vi "DelayProject_AirDelay.vi"() -> ()   [LabVIEW 2020]
uses:
  C:/DATA/Megan/LabviewScripts/ThorlabsKinesisDrivers/Thorlabs.MotionControl.Benchtop.BrushlessMotorCLI.dll
  Thorlabs.MotionControl.Benchtop.BrushlessMotorCLI.dll
  C:/DATA/Megan/LabviewScripts/ThorlabsKinesisDrivers/Thorlabs.MotionControl.Controls.dll
  Thorlabs.MotionControl.Controls.dll
  Program Files (x86)/National Instruments/LabVIEW 2011/user.lib/Nanonis Prog Interface/Nanonis Prog Interface.lvlib
panel:
  in  "Start Move B":bool
  in  "Set Position B (mm)":ext format="%.3f"
  in  "Clear Plots":bool
  in  "Data3":dbl[][](array[numeric])
  out "AFM":cluster{dbl[], dbl[]}[](graph)
  in  "Data2":dbl[][](array[numeric])
  in  "Data1":dbl[][](array[numeric])
  in  "Plot3":bool
  in  "Plot2":bool
  in  "Plot1":bool
  out "Optics":cluster{dbl[], dbl[]}[](graph)
  out "Array":string[][](array[string])
  in  "AC bias (Hz)":string
  in  "AC bias":string
  in  "DC bias":string
  in  "Tip lift":string
  in  "Time const":string
  in  "Prop gain":string
  in  "Polarization":string
  in  "Notes":string
  in  "Location":string
  out "AC bias (Hz)":string="AC Bias (Hz)"
  out "AC bias":string="AC Bias (V)"
  out "DC bias":string="DC Bias (V)"
  out "Polarization":string="Polarization (deg)"
  out "Tip Lift":string="Tip Lift"
  out "Notes":string="Notes"
  out "Location":string="Location"
  out "Time Const":string="Time constant (s)"
  out "Prop Gain":string="Proportional gain (m/Hz)"
  in  "Net Power":string
  in  "Wavelength":string
  out "Net Power":string="Net power (mW)"
  out "Wavelength":string="Wavelength (nm)"
  out "Instantaneous":dbl
  in  "Channel":dbl
  out "Average":dbl
  in  "Wait After (ms)":dbl=100.0
  in  "Wait Before (ms)":dbl=100.0
  in  "Points per Step":dbl=10.0
  in  "Save Sweep":bool
  out "Total Time (min:sec)":string
  out "Range (fs)":dbl
  out "Total Distance (mm)":dbl
  in  "Step Size (mm)":dbl format="%.4f"
  in  "Start Position (mm)":dbl=80.0
  in  "End Position (mm)":dbl=90.0
  out "Step Size (fs)":dbl=100.0
  out "Status":string
  in  "Set Position A (mm)":ext format="%.3f"
  in  "Start Move A":bool
  in  "Start Sweep":bool
  out "Time Remaining (min:sec)":string
  in  "Stop Sweep":bool
  out "Position  (mm)":ext format="%.3f"
  in  "BenchtopBrushlessControl":refnum<k24>(container)
  # "Air Delay"
  # "Sweep"
  # "This program moves the DSS022 translational delay stage either in a single step (Move), or a  stepped sweep (Sweep). \n\nThe sequence of events in the Sweep is as follows:\n1) Home the stage.\n2) Go to the Start Position; wait 1s.\n3) Move by Step Size.\n4)  Wait Before time. \n5) Write Position to Nanonis Output 8.\n6) Read all Nanonis Channels, Points per Step times.\n7) Take the average of these instantaneous readouts.\n8) Wait After time.\n9) Repeat 3-8 for each step. \n10) Save all Nanonis channels and record Attributes in header.\n\nThe Readouts are for this VI display only, to visualize what the program is doing. Channel is the Nanonis channel displayed. \n\nIf the Set/Start/End positions are outside of the operating range [50:210]mm, the Move/Sweep will not execute. Short wait times may lead to errors if  they don't allow time  to move. \n\nThis VI needs to be opened from the project directory. This project and VI need to be in the same directory as the Thorlabs Kinesis folder, and require a 64-bit version of Labview. This program cannot run simultaneously with WedgeDelay.vi"
  # "Attributes"
  # "Parameters"
  # "Readouts"
  # "Move A"
  # "Move B"
  # "Wedge Delay: 43mm"
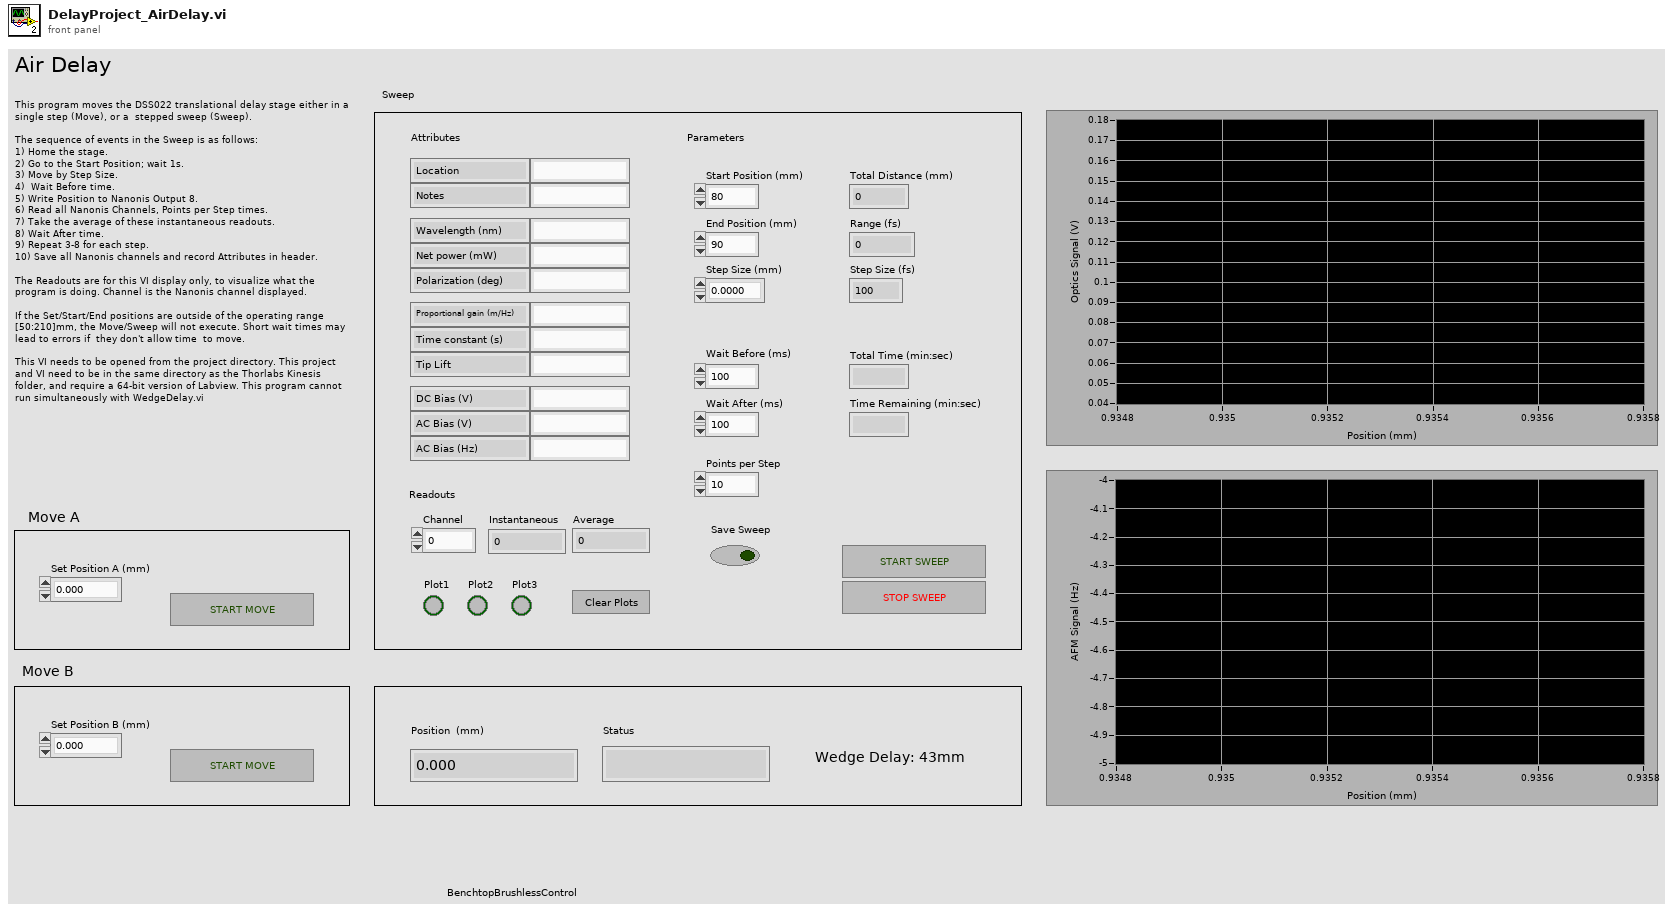
[diagram p1: front panel]
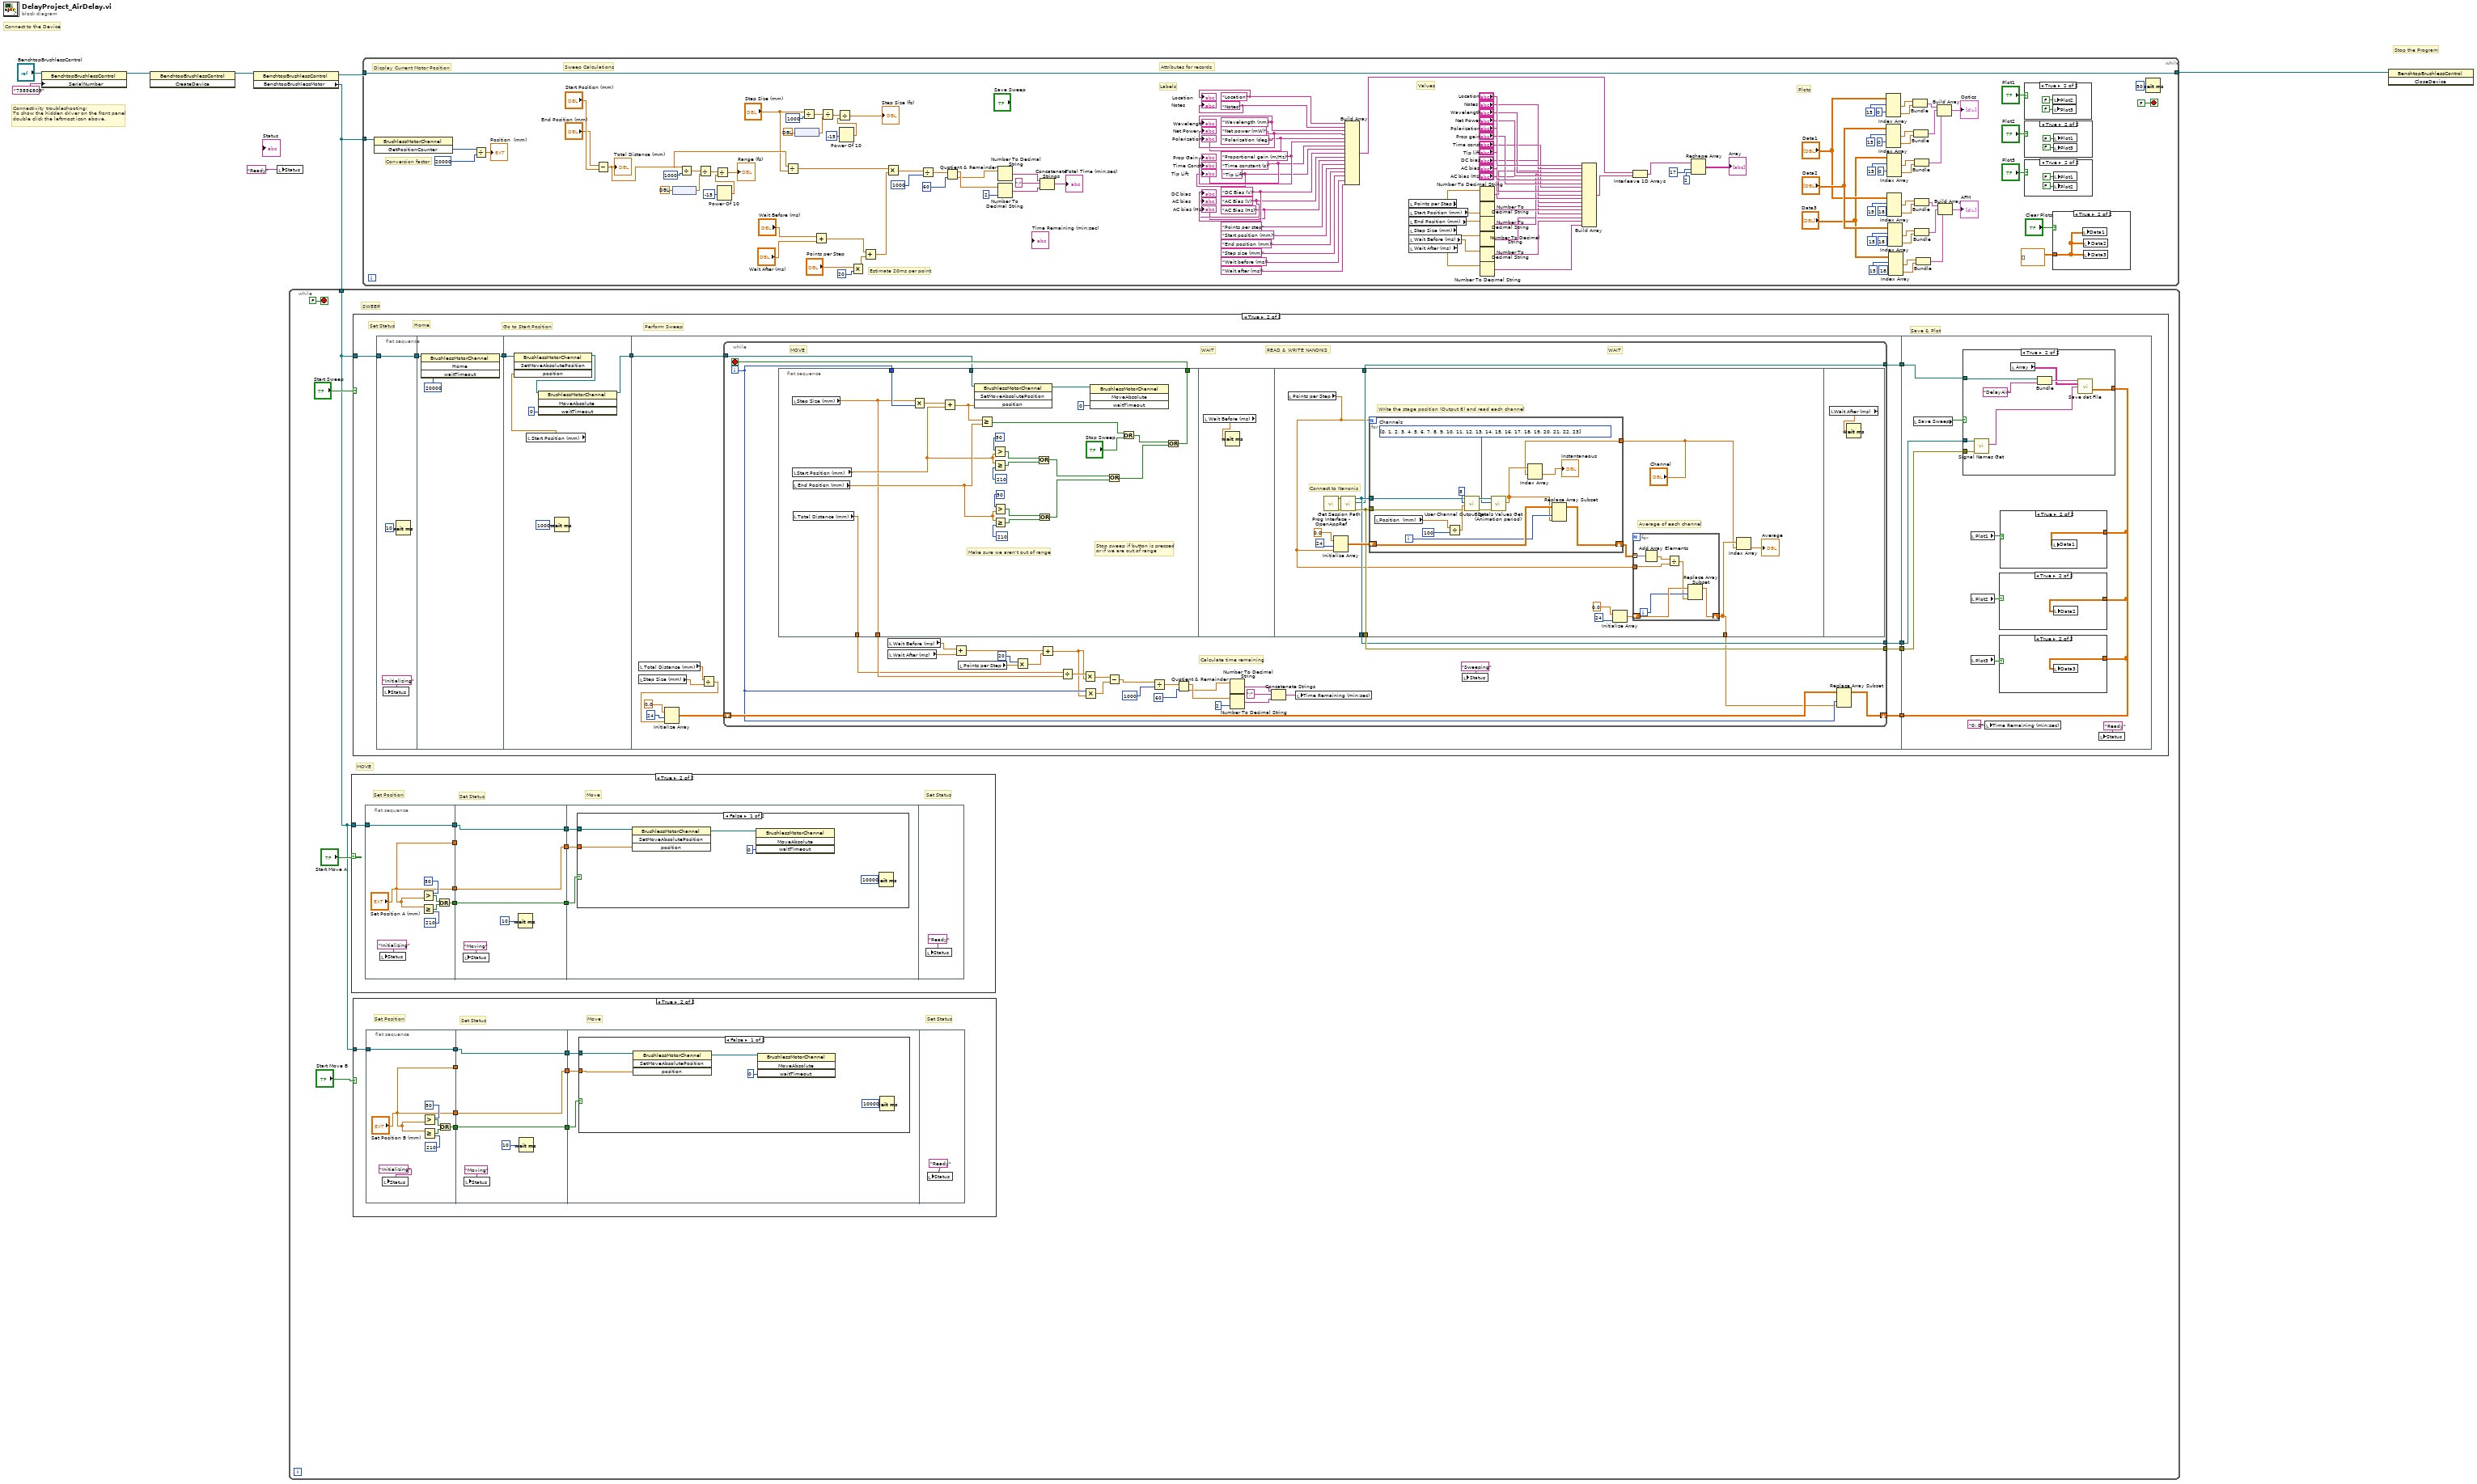
[diagram p0: block diagram]
diagram:
  # "Connectivity troubleshooting: \nTo show the hidden driver on the front panel \ndouble click the leftmost icon above."
  # "Stop the Program"
  # "Connect to the Device"
  n1 = property class="BenchtopBrushlessControl"(reference="BenchtopBrushlessControl", "SerialNumber"="73856809") -> (reference out=w7:refnum<k24>)  [unwired: 1 in, 1 out]
  n2 = invoke class="BenchtopBrushlessControl" method="CreateDevice"(reference=w7) -> (reference out=w4:refnum<k24>)  [unwired: 2 in, 2 out]
  n3 = property class="BenchtopBrushlessControl"(reference=w4) -> (reference out=w3:refnum<k24>, "BenchtopBrushlessMotor"=w2:refnum<k24>)  [unwired: 1 in, 1 out]
  n4 = local write "Status"("Ready") -> ()
  n5 = while {
    tunnel: w2 -> [w9]
    stop <- FALSE stop-if-true
    # "MOVE"
    # "SWEEP"
    n6 = case shown="True" "Start Move A" {
      tunnel: w9 -> [_ w51]
      frame False {
      }
      frame True {
        # "Set Status"
        # "Move"
        # "Set Status"
        # "Set Position"
        n7 = flat-sequence {
          tunnel: w51 -> [w59]
          tunnel: [w59] -> w50
          tunnel: ["Set Position A (mm)"] -> w49
          tunnel: [w53] -> w48
          tunnel: ["Set Position A (mm)"] -> w45
          tunnel: w50 -> [w62]
          tunnel: w49 -> [_]
          tunnel: w48 -> [w64]
          tunnel: [w64] -> w47
          tunnel: [w63] -> w46
          tunnel: w45 -> [w63]
          tunnel: [w62] -> w44
          tunnel: w47 -> [w67]
          tunnel: w46 -> [w66]
          tunnel: w44 -> [w65]
          frame #0 {
            n8 = local write "Status"("Initializing") -> ()
            n9 = Greater?(x=50, y="Set Position A (mm)") -> (0:w58:bool)
            n10 = Greater Or Equal?(x="Set Position A (mm)", y=210) -> (x >= y?=w57:bool)
            n11 = Or(x=w58, y=w57) -> (x .or. y?=w53:bool)
          }
          frame #1 {
            n12 = local write "Status"("Moving") -> ()
            n13 = Wait (ms)(milliseconds to wait=10) -> ()  [unwired: 1 out]
          }
          frame #2 {
            n14 = case shown="False" w67 {
              tunnel: w66 -> [w69 _]
              tunnel: w65 -> [w70 _]
              frame False {
                n15 = invoke class="BrushlessMotorChannel" method="SetMoveAbsolutePosition"(reference=w70, "position"=w69) -> (reference out=w72:refnum<k24>)  [unwired: 2 in, 3 out]
                n16 = invoke class="BrushlessMotorChannel" method="MoveAbsolute"(reference=w72, "waitTimeout"=0) -> ()  [unwired: 2 in, 4 out]
                n17 = Wait (ms)(milliseconds to wait=10000) -> ()  [unwired: 1 out]
              }
              frame True {
              }
            }
          }
          frame #3 {
            n18 = local write "Status"("Ready") -> ()
          }
        }
      }
    }
    n19 = case shown="True" "Start Move B" {
      tunnel: w9 -> [_ w21]
      frame False {
      }
      frame True {
        # "Set Status"
        # "Move"
        # "Set Status"
        # "Set Position"
        n20 = flat-sequence {
          tunnel: w21 -> [w29]
          tunnel: [w29] -> w20
          tunnel: ["Set Position B (mm)"] -> w19
          tunnel: [w24] -> w18
          tunnel: ["Set Position B (mm)"] -> w15
          tunnel: w20 -> [w32]
          tunnel: w19 -> [_]
          tunnel: w18 -> [w34]
          tunnel: [w34] -> w17
          tunnel: [w33] -> w16
          tunnel: w15 -> [w33]
          tunnel: [w32] -> w14
          tunnel: w17 -> [w37]
          tunnel: w16 -> [w36]
          tunnel: w14 -> [w35]
          frame #0 {
            n21 = local write "Status"("Initializing") -> ()
            n22 = Greater?(x=50, y="Set Position B (mm)") -> (0:w28:bool)
            n23 = Greater Or Equal?(x="Set Position B (mm)", y=210) -> (x >= y?=w27:bool)
            n24 = Or(x=w28, y=w27) -> (x .or. y?=w24:bool)
          }
          frame #1 {
            n25 = local write "Status"("Moving") -> ()
            n26 = Wait (ms)(milliseconds to wait=10) -> ()  [unwired: 1 out]
          }
          frame #2 {
            n27 = case shown="False" w37 {
              tunnel: w36 -> [w39 _]
              tunnel: w35 -> [w40 _]
              frame False {
                n28 = invoke class="BrushlessMotorChannel" method="SetMoveAbsolutePosition"(reference=w40, "position"=w39) -> (reference out=w42:refnum<k24>)  [unwired: 2 in, 3 out]
                n29 = invoke class="BrushlessMotorChannel" method="MoveAbsolute"(reference=w42, "waitTimeout"=0) -> ()  [unwired: 2 in, 4 out]
                n30 = Wait (ms)(milliseconds to wait=10000) -> ()  [unwired: 1 out]
              }
              frame True {
              }
            }
          }
          frame #3 {
            n31 = local write "Status"("Ready") -> ()
          }
        }
      }
    }
    n32 = case shown="True" "Start Sweep" {
      tunnel: w9 -> [_ w81]
      frame False {
      }
      frame True {
        # "Save & Plot"
        # "Set Status"
        # "Perform Sweep"
        # "Go to Start Position"
        # "Home"
        n33 = flat-sequence {
          tunnel: w81 -> [w84]
          tunnel: [w84] -> w80
          tunnel: [w85] -> w79
          tunnel: w80 -> [w87]
          tunnel: w79 -> [w93]
          tunnel: [w90] -> w78
          tunnel: w78 -> [w104]
          tunnel: [w103] -> w77
          tunnel: [w102] -> w76
          tunnel: [w101] -> w75
          tunnel: [w94] -> w74
          tunnel: w77 -> [w210]
          tunnel: w76 -> [w209]
          tunnel: w75 -> [w208]
          tunnel: w74 -> [w206]
          frame #0 {
            n34 = local write "Status"("Initializing") -> ()
            n35 = Wait (ms)(milliseconds to wait=10) -> ()  [unwired: 1 out]
          }
          frame #1 {
            n36 = invoke class="BrushlessMotorChannel" method="Home"(reference=w87, "waitTimeout"=20000) -> (reference out=w85:refnum<k24>)  [unwired: 2 in, 3 out]
          }
          frame #2 {
            n37 = local read "Start Position (mm)"() -> (w88:dbl)
            n38 = invoke class="BrushlessMotorChannel" method="SetMoveAbsolutePosition"(reference=w93, "position"=w88) -> (reference out=w91:refnum<k24>)  [unwired: 2 in, 3 out]
            n39 = invoke class="BrushlessMotorChannel" method="MoveAbsolute"(reference=w91, "waitTimeout"=0) -> (reference out=w90:refnum<k24>)  [unwired: 2 in, 3 out]
            n40 = Wait (ms)(milliseconds to wait=1000) -> ()  [unwired: 1 out]
          }
          frame #3 {
            n41 = local read "Step Size (mm)"() -> (w97:dbl)
            n42 = local read "Total Distance (mm)"() -> (w98:dbl)
            n43 = Divide(x=w98, y=w97) -> (x/y=w96:dbl)
            n44 = Initialize Array(0.0, 24, w96) -> (w95:dbl[][])
            n45 = while {
              tunnel: w104 -> [w136]
              tunnel: [w116] -> w103
              tunnel: [w117] -> w102
              tunnel: [w115] -> w101
              shift-right: [w111] -> w94
              shift-left: w95 -> [w114]
              i -> [w113]
              stop <- w137 stop-if-true
              # "WAIT"
              # "READ & WRITE NANONIS"
              # "WAIT"
              # "MOVE"
              # "Calculate time remaining"
              n46 = flat-sequence {
                tunnel: w113 -> [w142]
                tunnel: [w141] -> w137
                tunnel: w136 -> [w140]
                tunnel: [w139] -> w126
                tunnel: [w138] -> w125
                tunnel: [w169] -> w117
                tunnel: [w168] -> w116
                tunnel: [w167] -> w115
                tunnel: [w166] -> w112
                frame #0 {
                  # "Stop sweep if button is pressed\nor if we are out of range"
                  # "Make sure we aren't out of range"
                  n47 = local read "Step Size (mm)"() -> (w139:dbl)
                  n48 = local read "Start Position (mm)"() -> (w161:dbl)
                  n49 = local read "End Position (mm)"() -> (w162:dbl)
                  n50 = local read "Total Distance (mm)"() -> (w138:dbl)
                  n51 = Multiply(x=w139, y=w142) -> (x*y=w147:dbl)
                  n52 = Add(x=w147, y=w161) -> (x+y=w148:dbl)
                  n53 = invoke class="BrushlessMotorChannel" method="SetMoveAbsolutePosition"(reference=w140, "position"=w148) -> (reference out=w143:refnum<k24>)  [unwired: 2 in, 3 out]
                  n54 = Greater Or Equal?(x=w148, y=w162) -> (x >= y?=w146:bool)
                  n55 = Greater?(x=50, y=w161) -> (0:w153:bool)
                  n56 = Greater Or Equal?(x=w161, y=210) -> (x >= y?=w154:bool)
                  n57 = Greater?(x=50, y=w162) -> (0:w157:bool)
                  n58 = Greater Or Equal?(x=w162, y=210) -> (x >= y?=w158:bool)
                  n59 = Or(x=w153, y=w154) -> (x .or. y?=w159:bool)
                  n60 = Or(x=w157, y=w158) -> (x .or. y?=w160:bool)
                  n61 = invoke class="BrushlessMotorChannel" method="MoveAbsolute"(reference=w143, "waitTimeout"=0) -> ()  [unwired: 2 in, 4 out]
                  n62 = Or(x=w159, y=w160) -> (x .or. y?=w150:bool)
                  n63 = Or(x=w146, y="Stop Sweep") -> (x .or. y?=w149:bool)
                  n64 = Or(x=w149, y=w150) -> (x .or. y?=w141:bool)
                }
                frame #1 {
                  n65 = local read "Wait Before (ms)"() -> (w163:dbl)
                  n66 = Wait (ms)(milliseconds to wait=w163) -> ()  [unwired: 1 out]
                }
                frame #2 {
                  # "Write the stage position (Output 8) and read each channel"
                  # "Average of each channel"
                  # "Connect to Nanonis"
                  n67 = local read "Points per Step"() -> (w165:dbl)
                  n68 = call "Prog Interface - OpenAppRef.vi"() -> ("Error out"=w170:errorcluster, "Application reference"=w171:refnum<vi>)  [unwired: 6 in]
                  n69 = Initialize Array(0.0, 24, w165) -> (w174:dbl[][])
                  n70 = call "Get Session Path.vi"("error in (no error)"=w170, "Application ref in"=w171) -> ("error out"=w169:errorcluster, "Session path"=w167:path, "Application ref out"=w168:refnum<vi>)  [unwired: 7 in]
                  n71 = for {
                    N: w165 -> [_]
                    tunnel: w169 -> [w195]
                    tunnel: w168 -> [w194]
                    shift-right: [w193] -> w178
                    shift-left: w174 -> [w192]
                    tunnel: "Channel" -> [w187]
                    i -> [w191]
                    w188 = i32[] [0, 1, 2, 3, 4, 5, 6, 7, 8, 9, 10, 11, 12, 13, 14, 15, 16, 17, 18, 19, 20, 21, 22, 23]  # Channels
                    n72 = local read "Position  (mm)"() -> (w189:ext)
                    n73 = Divide(x=w189, y=100) -> (x/y=w198:ext)
                    n74 = call "User Channel Output Set.vi"("error in (no error)"=w195, "Output value (physical unit)"=w198, "User output channel (1-8)"=8, "Application ref in"=w194) -> ("error out"=w200:errorcluster, "Application ref out"=w199:refnum<vi>)  [unwired: 5 in]
                    n75 = call "Signals Values Get (Animation period).vi"("error in (no error)"=w200, "Signals indexes (0-23)"=w188, "Application ref in"=w199) -> ("Signals Values"=w190:sgl[])  [unwired: 5 in, 2 out]
                    n76 = Index Array(array=w190, index #1=w187) -> (element #1=→"Instantaneous":sgl)  [unwired: 1 in, 1 out]
                    n77 = Replace Array Subset(array=w192, new element=w190, index (col)=w191) -> (w193:dbl[][])  [unwired: 1 in]
                  }
                  n78 = Initialize Array(0.0, 24) -> (w177:dbl[])
                  n79 = for {
                    tunnel: w165 -> [w186]
                    tunnel: w178 -> [w182] mode=indexing
                    shift-right: [w184] -> w166
                    shift-left: w177 -> [w185]
                    i -> [w183]
                    n80 = Add Array Elements(numeric array=w182) -> (sum=w180:dbl)
                    n81 = Divide(x=w180, y=w186) -> (x/y=w181:dbl)
                    n82 = Replace Array Subset(array=w185, new element=w181, index=w183) -> (w184:dbl[])
                  }
                  n83 = Index Array(array=w166, index="Channel") -> (element=→"Average":dbl)
                }
                frame #3 {
                  n84 = local read "Wait After (ms)"() -> (w202:dbl)
                  n85 = Wait (ms)(milliseconds to wait=w202) -> ()  [unwired: 1 out]
                }
              }
              n86 = local read "Wait Before (ms)"() -> (w119:dbl)
              n87 = local read "Wait After (ms)"() -> (w118:dbl)
              n88 = Add(x=w119, y=w118) -> (x+y=w109:dbl)
              n89 = local read "Points per Step"() -> (w110:dbl)
              n90 = Multiply(x=20, y=w110) -> (x*y=w107:dbl)
              n91 = Add(x=w109, y=w107) -> (x+y=w108:dbl)
              n92 = Divide(x=w125, y=w126) -> (x/y=w127:dbl)
              n93 = Multiply(x=w127, y=w108) -> (x*y=w128:dbl)
              n94 = Multiply(x=w113, y=w108) -> (x*y=w130:dbl)
              n95 = Subtract(x=w128, y=w130) -> (x-y=w129:dbl)
              n96 = Divide(x=w129, y=1000) -> (x/y=w135:dbl)
              n97 = Quotient & Remainder(x=w135, y=60) -> (x-y*floor(x/y)=w134:dbl, floor(x/y)=w133:dbl)
              n98 = Number To Decimal String(number=w133) -> (decimal integer string=w132:string)  [unwired: 1 in]
              n99 = Number To Decimal String(number=w134, width (-)=2) -> (decimal integer string=w131:string)
              n100 = Concatenate Strings(w132, ":", w131) -> (w105:string)
              n101 = local write "Time Remaining (min:sec)"(w105) -> ()
              n102 = local write "Status"("Sweeping") -> ()
              n103 = Replace Array Subset(array=w114, new element=w112, index (col)=w113) -> (w111:dbl[][])  [unwired: 1 in]
            }
          }
          frame #4 {
            n104 = local read "Save Sweep"() -> (w211:bool)
            n105 = case shown="True" w211 {
              tunnel: w209 -> [_ w221]
              tunnel: w210 -> [_ w220]
              tunnel: w208 -> [_ w218]
              tunnel: w206 -> [_ w217]
              frame False {
              }
              frame True {
                n106 = call "Signal Names Get.vi"("error in (no error)"=w221, "Application ref in"=w220) -> ("Signals Names"=w219:string[])  [unwired: 5 in, 2 out]
                n107 = local read "Array"() -> (w216:string[][])
                n108 = Bundle("Session path"=w218, "DelayAir") -> (w223:cluster{"Session path":path, string})  [unwired: 1 in]
                n109 = call "Save dat File.vi"("Filename control"=w223, "Attributes"=w216, "Channels names"=w219, "Data"=w217) -> ()  [unwired: 8 in, 4 out]
              }
            }
            n110 = local read "Plot1"() -> (w203:bool)
            n111 = local read "Plot2"() -> (w204:bool)
            n112 = local read "Plot3"() -> (w205:bool)
            n113 = local write "Time Remaining (min:sec)"("0: 0") -> ()
            n114 = case shown="True" w204 {
              tunnel: w206 -> [_ w214]
              frame False {
              }
              frame True {
                n115 = local write "Data2"(w214) -> ()
              }
            }
            n116 = case shown="True" w205 {
              tunnel: w206 -> [_ w213]
              frame False {
              }
              frame True {
                n117 = local write "Data3"(w213) -> ()
              }
            }
            n118 = case shown="True" w203 {
              tunnel: w206 -> [_ w215]
              frame False {
              }
              frame True {
                n119 = local write "Data1"(w215) -> ()
              }
            }
            n120 = local write "Status"("Ready") -> ()
          }
        }
      }
    }
  }
  n121 = while {
    tunnel: [w355] -> w6
    tunnel: w3 -> [w355]
    tunnel: w2 -> [w354]
    stop <- FALSE stop-if-true
    w277 = "Polarization (deg)"
    w280 = "Notes"
    w281 = "Location"
    w274 = "Tip Lift"
    w271 = "AC Bias (Hz)"
    w272 = "AC Bias (V)"
    w273 = "DC Bias (V)"
    w275 = "Time constant (s)"
    w276 = "Proportional gain (m/Hz)"
    w278 = "Net power (mW)"
    w279 = "Wavelength (nm)"
    # "Plots"
    # "Estimate 20ms per point"
    # "Values"
    # "Labels"
    # "Attributes for records"
    # "Sweep Calculations"
    # "Display Current Motor Position"
    # "Conversion factor"
    n122 = invoke class="BrushlessMotorChannel" method="GetPositionCounter"(reference=w354) -> ("GetPositionCounter"=w353:i32)  [unwired: 2 in, 2 out]
    n123 = Divide(x=w353, y=20000) -> (x/y=→"Position  (mm)":dbl)
    n124 = Subtract(x="End Position (mm)", y="Start Position (mm)") -> (x-y=w321:dbl)
    "Total Distance (mm)" <- w321
    n125 = node(ext[unit] 299792458.0) -> (w337:ext)
    n126 = Divide(x=w321, y=1000) -> (x/y=w338:dbl)
    n127 = Divide(x=w338, y=w337) -> (x/y=w336:ext)
    n128 = Power Of 10(x=-15) -> (10^x=w333:dbl)
    n129 = Divide(x=w336, y=w333) -> (x/y=→"Range (fs)":ext)
    n130 = Divide(x=w321, y="Step Size (mm)") -> (x/y=w318:dbl)
    n131 = node(ext[unit] 299792458.0) -> (w347:ext)
    n132 = Divide(x="Step Size (mm)", y=1000) -> (x/y=w346:dbl)
    n133 = Add(x="Wait Before (ms)", y="Wait After (ms)") -> (x+y=w269:dbl)
    n134 = Divide(x=w346, y=w347) -> (x/y=w348:ext)
    n135 = Power Of 10(x=-15) -> (10^x=w349:dbl)
    n136 = Divide(x=w348, y=w349) -> (x/y=→"Step Size (fs)":ext)
    n137 = Multiply(x="Points per Step", y=20) -> (x*y=w270:dbl)
    n138 = Add(x=w269, y=w270) -> (x+y=w268:dbl)
    n139 = Multiply(x=w318, y=w268) -> (x*y=w322:dbl)
    n140 = Divide(x=w322, y=1000) -> (x/y=w330:dbl)
    n141 = Quotient & Remainder(x=w330, y=60) -> (x-y*floor(x/y)=w328:dbl, floor(x/y)=w327:dbl)
    n142 = Number To Decimal String(number=w327) -> (decimal integer string=w326:string)  [unwired: 1 in]
    n143 = Number To Decimal String(number=w328, width (-)=2) -> (decimal integer string=w324:string)
    n144 = Concatenate Strings(w326, ":", w324) -> (→"Total Time (min:sec)":string)
    n145 = Build Array(w281, w280, w279, w278, w277, w276, w275, w274, w273, w272, w271, "Points per step", "Start position (mm)", "End position (mm)", "Step size (mm)", "Wait before (ms)", "Wait after (ms)") -> (w285:string[])
    n146 = local read "Points per Step"() -> (w315:dbl)
    n147 = local read "Start Position (mm)"() -> (w314:dbl)
    n148 = local read "End Position (mm)"() -> (w313:dbl)
    n149 = local read "Step Size (mm)"() -> (w312:dbl)
    n150 = local read "Wait Before (ms)"() -> (w311:dbl)
    n151 = local read "Wait After (ms)"() -> (w310:dbl)
    n152 = Number To Decimal String(number=w315) -> (decimal integer string=w297:string)  [unwired: 1 in]
    n153 = Number To Decimal String(number=w314) -> (decimal integer string=w296:string)  [unwired: 1 in]
    n154 = Number To Decimal String(number=w313) -> (decimal integer string=w295:string)  [unwired: 1 in]
    n155 = Number To Decimal String(number=w312) -> (decimal integer string=w294:string)  [unwired: 1 in]
    n156 = Number To Decimal String(number=w311) -> (decimal integer string=w293:string)  [unwired: 1 in]
    n157 = Number To Decimal String(number=w310) -> (decimal integer string=w286:string)  [unwired: 1 in]
    n158 = Build Array("Location", "Notes", "Wavelength", "Net Power", "Polarization", "Prop gain", "Time const", "Tip lift", "DC bias", "AC bias", "AC bias (Hz)", w297, w296, w295, w294, w293, w286) -> (w284:string[])
    n159 = Interleave 1D Arrays(w285, w284) -> (w283:string[])
    n160 = Reshape Array(w283, 17, 2) -> (→"Array":string[][])
    n161 = Index Array(array="Data1", index (row) #1=15, index (row) #2=0) -> (element #1=w262:dbl[], element #2=w263:dbl[])  [unwired: 2 in]
    n162 = Index Array(array="Data2", index (row) #1=15, index (row) #2=0) -> (element #1=w257:dbl[], element #2=w258:dbl[])  [unwired: 2 in]
    n163 = Index Array(array="Data3", index (row) #1=15, index (row) #2=0) -> (element #1=w253:dbl[], element #2=w254:dbl[])  [unwired: 2 in]
    n164 = Index Array(array="Data1", index (row) #1=15, index (row) #2=18) -> (element #1=w246:dbl[], element #2=w247:dbl[])  [unwired: 2 in]
    n165 = Index Array(array="Data2", index (row) #1=15, index (row) #2=18) -> (element #1=w242:dbl[], element #2=w243:dbl[])  [unwired: 2 in]
    n166 = Index Array(array="Data3", index (row) #1=15, index (row) #2=18) -> (element #1=w238:dbl[], element #2=w239:dbl[])  [unwired: 2 in]
    n167 = Bundle("Data1"=w262, "Data1"=w263) -> (w250:cluster{"Data1":dbl[], "Data1":dbl[]})  [unwired: 1 in]
    n168 = Bundle("Data2"=w257, "Data2"=w258) -> (w249:cluster{"Data2":dbl[], "Data2":dbl[]})  [unwired: 1 in]
    n169 = Bundle("Data3"=w253, "Data3"=w254) -> (w248:cluster{"Data3":dbl[], "Data3":dbl[]})  [unwired: 1 in]
    n170 = Bundle("Data1"=w246, "Data1"=w247) -> (w235:cluster{"Data1":dbl[], "Data1":dbl[]})  [unwired: 1 in]
    n171 = Bundle("Data2"=w242, "Data2"=w243) -> (w234:cluster{"Data2":dbl[], "Data2":dbl[]})  [unwired: 1 in]
    n172 = Bundle("Data3"=w238, "Data3"=w239) -> (w233:cluster{"Data3":dbl[], "Data3":dbl[]})  [unwired: 1 in]
    n173 = Build Array(w250, w249, w248) -> (→"Optics":cluster{"Data3":dbl[], "Data3":dbl[]}[])
    n174 = Build Array(w235, w234, w233) -> (→"AFM":cluster{"Data3":dbl[], "Data3":dbl[]}[])
    n175 = case shown="True" "Plot1" {
      frame False {
      }
      frame True {
        n176 = local write "Plot2"(FALSE) -> ()
        n177 = local write "Plot3"(FALSE) -> ()
      }
    }
    n178 = case shown="True" "Plot2" {
      frame False {
      }
      frame True {
        n179 = local write "Plot1"(FALSE) -> ()
        n180 = local write "Plot3"(FALSE) -> ()
      }
    }
    n181 = case shown="True" "Plot3" {
      frame False {
      }
      frame True {
        n182 = local write "Plot1"(FALSE) -> ()
        n183 = local write "Plot2"(FALSE) -> ()
      }
    }
    n184 = case shown="True" "Clear Plots" {
      tunnel: dbl[][] [] ("Plot 3") -> [_ w362]
      frame False {
      }
      frame True {
        n185 = local write "Data1"(w362) -> ()
        n186 = local write "Data2"(w362) -> ()
        n187 = local write "Data3"(w362) -> ()
      }
    }
    n188 = Wait (ms)(milliseconds to wait=50) -> ()  [unwired: 1 out]
    "Wavelength" <- w279
    "Net Power" <- w278
    "Prop Gain" <- w276
    "Time Const" <- w275
    "Location" <- w281
    "Notes" <- w280
    "Tip Lift" <- w274
    "Polarization" <- w277
    "DC bias" <- w273
    "AC bias" <- w272
    "AC bias (Hz)" <- w271
  }
  n189 = invoke class="BenchtopBrushlessControl" method="CloseDevice"(reference=w6) -> ()  [unwired: 2 in, 3 out]
